vi "Update Active Room Details.vi"(0 "Rooms Manager UI in":refnum<class "Rooms Manager UI.lvclass">, 5 "Room Size":string, 7 "Status":T1, 9 "Guest Name":string, 11 "error in (no error)":errorcluster, 12 "Contact Number":string, 13 "Count":string) -> (4 "Rooms Manager UI out":refnum<class "Rooms Manager UI.lvclass">, 15 "error out":errorcluster)   [LabVIEW 2023, in "Rooms Manager UI.lvlib" / "Rooms Manager UI.lvclass"]
uses:
  Rooms Manager UI.lvclass
  Central Data Manager/Central Data Manager/Room Occupancy Status.ctl
  Rooms Manager UI.lvclass/Rooms Manager UI.ctl
  Central Data Manager/Central Data Manager/Central Data Manager.lvclass
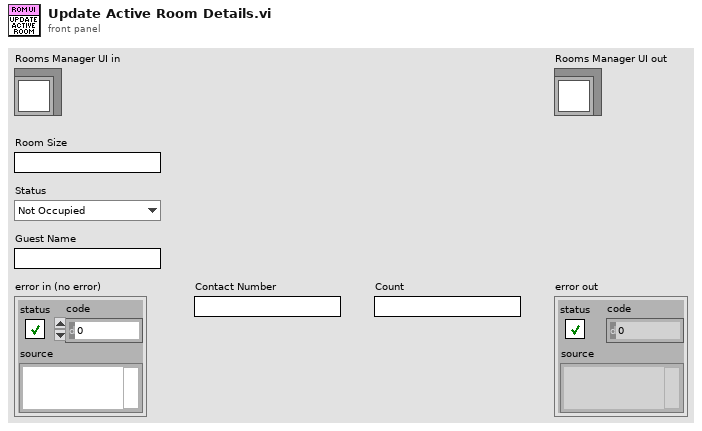
[diagram p1: front panel]
types:
  T1 = typedef "Central Data Manager.lvlib/Central Data Manager.lvclass/Room Occupancy Status.ctl" = enum16{"Not Occupied", "Occupied", "Under Maintainance", "Not Servicable"}
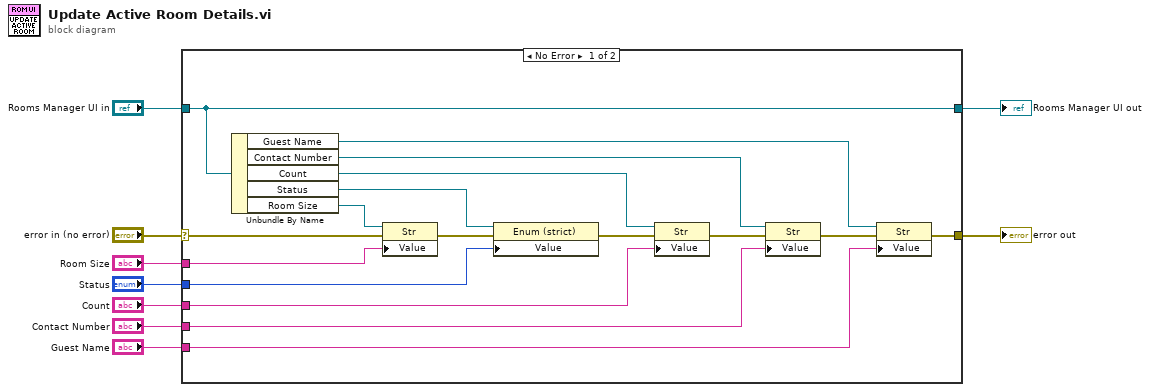
[diagram p0: block diagram]
diagram:
  n1 = case shown="No Error" "error in (no error)" {
    selector: "error in (no error)" -> [w22 w28]
    tunnel: [w21 w28] -> w8
    tunnel: [w20 w27] -> w6
    tunnel: "Rooms Manager UI in" -> [w20 w27]
    tunnel: "Guest Name" -> [w14 _]
    tunnel: "Contact Number" -> [w13 _]
    tunnel: "Count" -> [w12 _]
    tunnel: "Status" -> [w11 _]
    tunnel: "Room Size" -> [w10 _]
    frame No Error {
      n2 = Unbundle By Name(w20) -> ("Guest Name"=w15:refnum<vi>, "Contact Number"=w16:refnum<vi>, "Count"=w17:refnum<vi>, "Status"=w18:refnum<vi>, "Room Size"=w19:refnum<vi>)
      n3 = property class="Str"(reference=w19, error in=w22, "Value"=w10) -> (error out=w26:errorcluster)  [unwired: 1 out]
      n4 = property class="Enum (strict)"(reference=w18, error in=w26, "Value"=w11) -> (error out=w25:errorcluster)  [unwired: 1 out]
      n5 = property class="Str"(reference=w17, error in=w25, "Value"=w12) -> (error out=w24:errorcluster)  [unwired: 1 out]
      n6 = property class="Str"(reference=w16, error in=w24, "Value"=w13) -> (error out=w23:errorcluster)  [unwired: 1 out]
      n7 = property class="Str"(reference=w15, error in=w23, "Value"=w14) -> (error out=w21:errorcluster)  [unwired: 1 out]
    }
    frame Error {
    }
  }
  "error out" <- w8
  "Rooms Manager UI out" <- w6
